vi "Settings Dialog.vi"(8 "error in (no error)":errorcluster, 11 "Settings in":T2={"Hardware Configuration"={"DAQmx Input"="", "Max Input"=10.0, "Min Input"=-10.0, "Sample Rate"=1000.0, "DAQmx Task"=""}, "Logging Configuration"={"Log File Base Path"=path "", "TDMS File Reference"=refnum, "Channel names"=[], "Author"="", "Description"=""}}) -> (0 "error out":errorcluster, 1 "Cancelled?":bool=TRUE, 2 "UI Refresh Needed?":bool, 3 "Settings out":T2={"Hardware Configuration"={"DAQmx Input"="", "Max Input"=10.0, "Min Input"=-10.0, "Sample Rate"=1000.0, "DAQmx Task"=""}, "Logging Configuration"={"Log File Base Path"=path "C:/Users/jpassiak/Documents/LabVIEW Data/Logged Data.tdms", "TDMS File Reference"=refnum, "Channel names"=[], "Author"="", "Description"=""}})   [LabVIEW 2016, in "Settings.lvlib"]
doc: "Dialog for selecting user specified settings."
uses:
  Settings.lvlib
  Acquisition/Hardware Configuration.ctl
  <vilib>/Utility/xml.llb/Write to XML File(string).vi
  Acquisition/Acquisition.lvlib
panel:
  in  "Channel Names":string[](array[string])
  in  "Author":string
  in  "Description":string
  in  "Sample Rate (Hz)":dbl=1000.0 min=0.0 max=50000.0 step=1.0
  in  "Min Input (V)":dbl=-10.0 min=-10.0 max=10.0 step=0.1
  in  "Max Input (V)":dbl=10.0 min=-10.0 max=10.0 step=0.1
  in  "Acquisition channels":tag="Dev1/ai0"
  in  "Log File Path":path
  in  "Cancel Button":bool
  in  "OK Button":bool
  # "Non visible portion of dialog (needed for connector pane)."
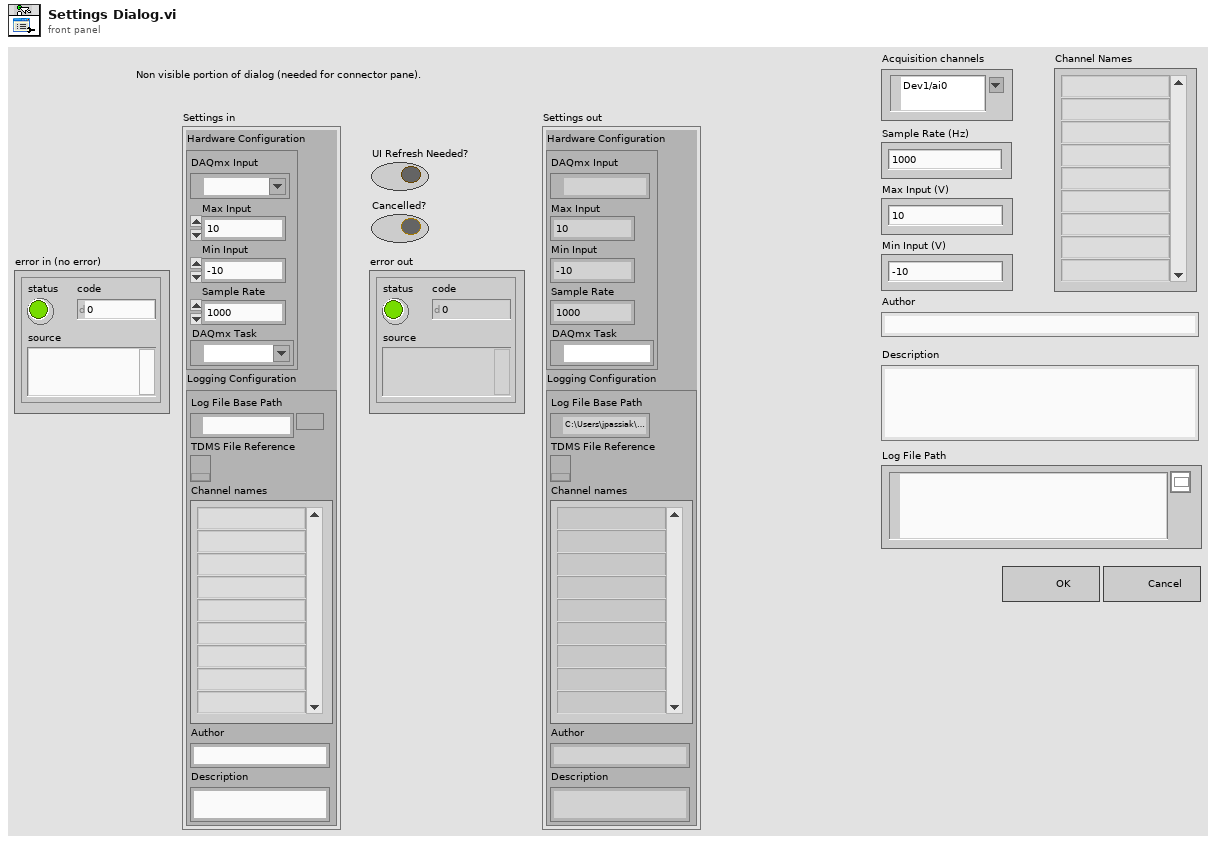
[diagram p1: front panel]
types:
  T1 = typedef "Acquisition.lvlib/Hardware Configuration.ctl" = cluster{"DAQmx Input":tag, "Max Input":dbl, "Min Input":dbl, "Sample Rate":dbl, "DAQmx Task":refnum<k21>}
  T2 = cluster{"Hardware Configuration":T1, "Logging Configuration":cluster{"Log File Base Path":path, "TDMS File Reference":refnum<k34>, "Channel names":string[], "Author":string, "Description":string}}
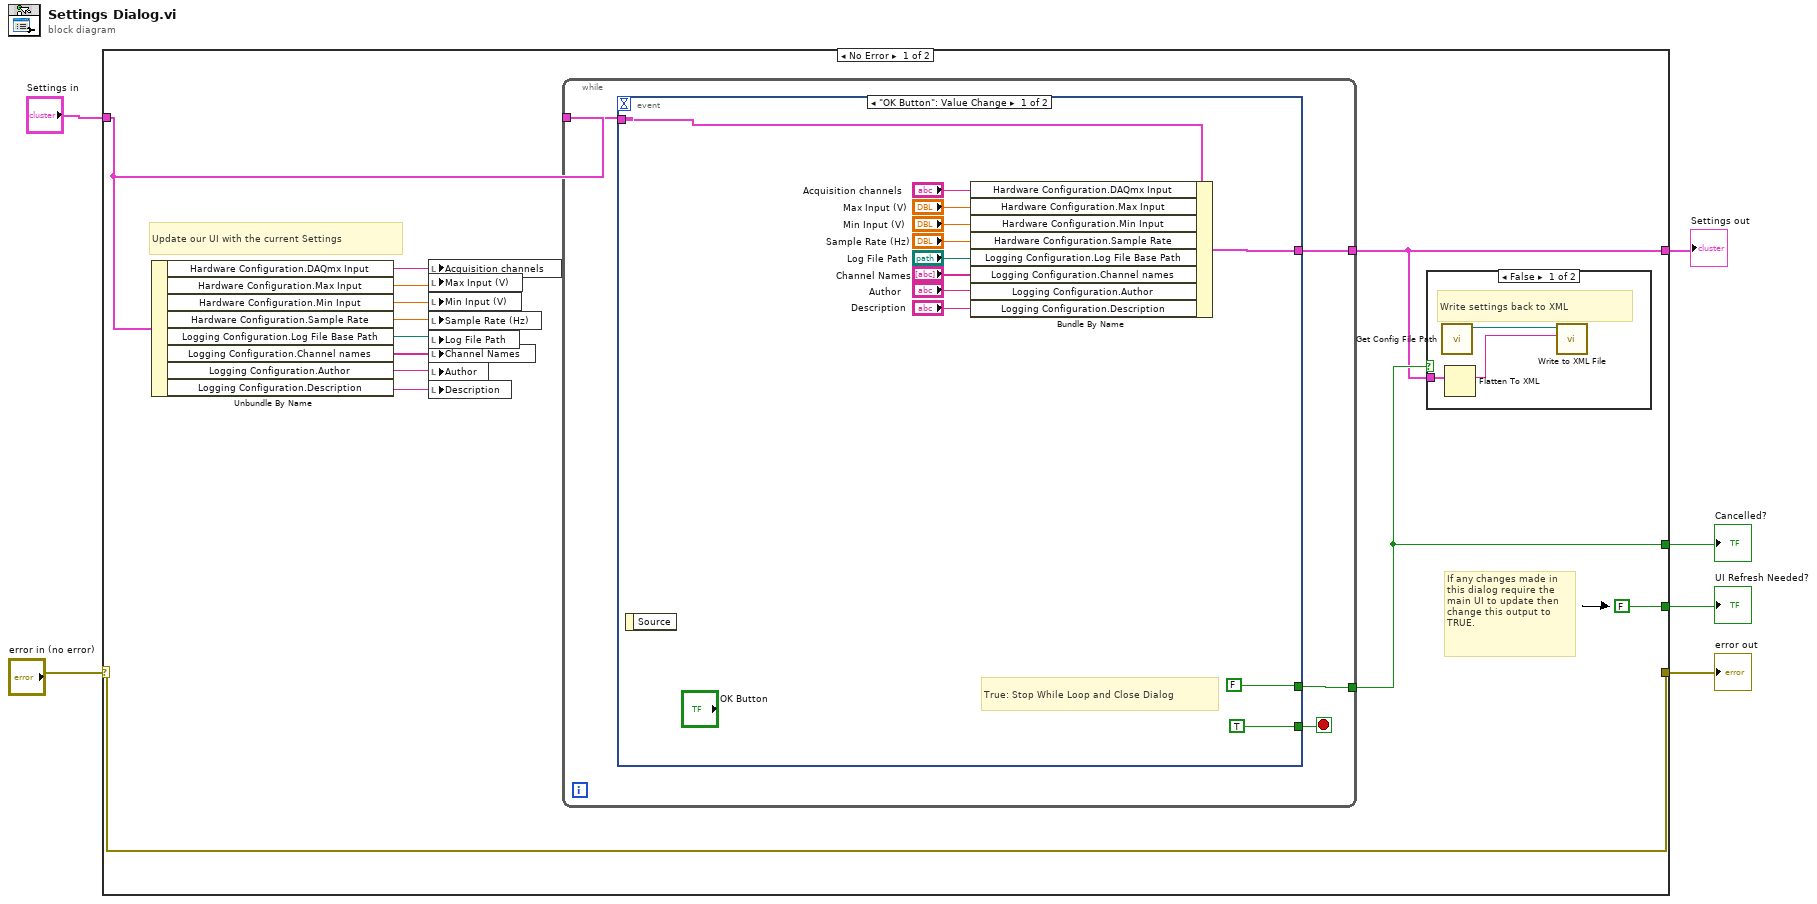
[diagram p0: block diagram]
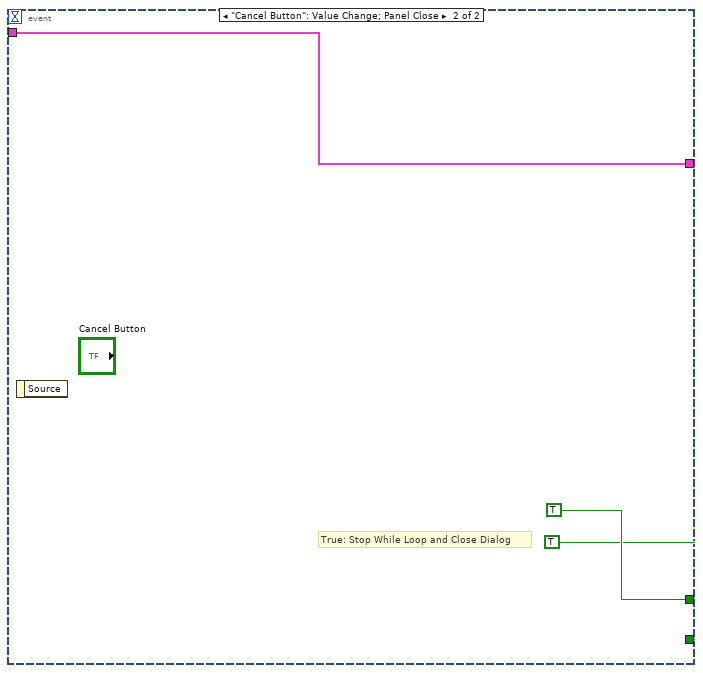
[diagram p2: hidden frame]
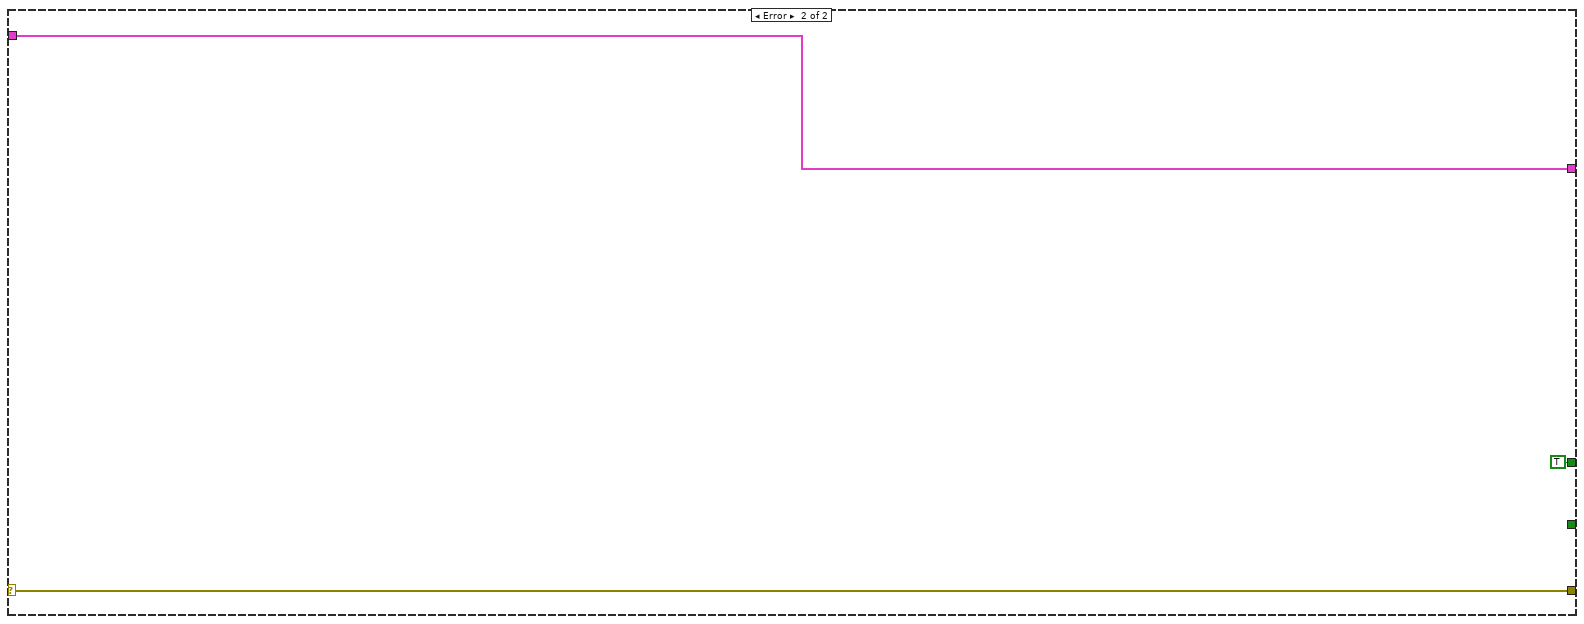
[diagram p4: hidden frame]
diagram:
  n1 = case shown="No Error" "error in (no error)" {
    selector: "error in (no error)" -> [w19 w44]
    tunnel: [w19 w44] -> w6
    tunnel: "Settings in" -> [w10 w43]
    tunnel: [w16 w43] -> w1
    tunnel: [FALSE ("UI Refresh Needed?") _] -> w5
    tunnel: [w17 TRUE ("UI Refresh Needed?")] -> w4
    frame No Error {
      # "Update our UI with the current Settings"
      # "If any changes made in this dialog require the main UI to update then change this output to TRUE."
      n2 = Unbundle By Name(w10) -> ("Hardware Configuration.DAQmx Input"=w12:tag, "Hardware Configuration.Max Input"=w13:dbl, "Hardware Configuration.Min Input"=w14:dbl, "Hardware Configuration.Sample Rate"=w15:dbl, "Logging Configuration.Log File Base Path"=w11:path, "Logging Configuration.Channel names"=w9:string[], "Logging Configuration.Author"=w8:string, "Logging Configuration.Description"=w7:string)
      n3 = local write "Acquisition channels"(w12) -> ()
      n4 = local write "Max Input (V)"(w13) -> ()
      n5 = local write "Min Input (V)"(w14) -> ()
      n6 = local write "Sample Rate (Hz)"(w15) -> ()
      n7 = local write "Log File Path"(w11) -> ()
      n8 = local write "Channel Names"(w9) -> ()
      n9 = local write "Author"(w8) -> ()
      n10 = local write "Description"(w7) -> ()
      n11 = while {
        tunnel: [w23] -> w17
        tunnel: [w22] -> w16
        tunnel: w10 -> [w21]
        stop <- w20 stop-if-true
        n12 = event shown="[0] \"OK Button\": Value Change" {
          selector: _ -> [_ _]
          dyn-events: _ -> [_ _]
          timeout: _ -> [_ _]
          tunnel: [w33 w38] -> w22
          tunnel: w21 -> [w32 w38]
          tunnel: [FALSE ("UI Refresh Needed?") TRUE ("UI Refresh Needed?")] -> w23
          tunnel: [TRUE TRUE] -> w20
          event "OK Button": Value Change {
            # "True: Stop While Loop and Close Dialog"
            n13 = event-data() -> ()  [unwired: 1 in, 1 out]
            n14 = Bundle By Name(cluster=w32, "Hardware Configuration.DAQmx Input"="Acquisition channels", "Hardware Configuration.Max Input"="Max Input (V)", "Hardware Configuration.Min Input"="Min Input (V)", "Hardware Configuration.Sample Rate"="Sample Rate (Hz)", "Logging Configuration.Log File Base Path"="Log File Path", "Logging Configuration.Channel names"="Channel Names", "Logging Configuration.Author"="Author", "Logging Configuration.Description"="Description") -> (w33:T2)
          }
          event "Cancel Button": Value Change; Panel Close {
            # "True: Stop While Loop and Close Dialog"
            n15 = event-data() -> ()  [unwired: 1 in, 1 out]
          }
        }
      }
      n16 = case shown="False" w17 {
        tunnel: w16 -> [w40 _]
        frame False {
          # "Write settings back to XML"
          n17 = call "Get Config File Path.vi"() -> ("XML File Path"=w41:path)  [unwired: 10 in, 1 out]
          n18 = Flatten To XML(anything=w40) -> (xml string=w39:string)
          n19 = call-poly <vilib>:"Write to XML File.vi"("XML Input"=w39, "XML File Path"=w41) -> ()  [unwired: 7 in, 3 out]
        }
        frame True {
        }
      }
    }
    frame Error {
    }
  }
  "UI Refresh Needed?" <- w5
  "error out" <- w6
  "Settings out" <- w1
  "Cancelled?" <- w4
